vi "getDeviceCount.vi"(11 "driver":string) -> (3 "device count":i32)   [LabVIEW 2015]
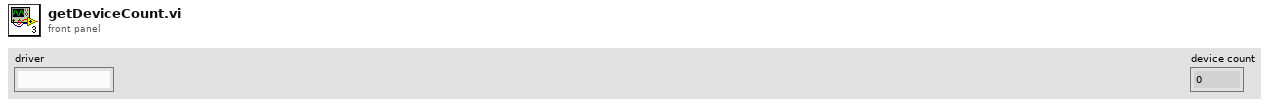
[diagram p1: front panel]
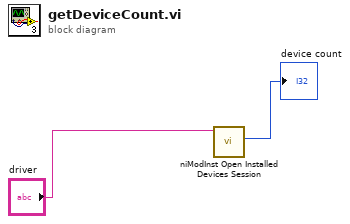
[diagram p0: block diagram]
diagram:
  n1 = call <instrlib>:"niModInst Open Installed Devices Session.vi"("driver"="driver") -> ("device count"=→"device count":i32)  [unwired: 8 in, 2 out]
